vi "etlUSBClose.vi"(1 "lens":enum16{"0", "1"}(ring)) -> ()   [LabVIEW 2017]
uses:
  globalDevices.vi
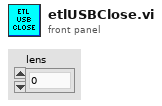
[diagram p1: front panel]
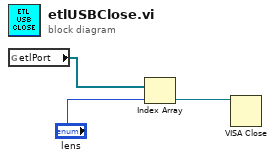
[diagram p0: block diagram]
diagram:
  n1 = global read "globalDevices.vi" "etlPort"() -> (w3:refnum<visa-resource-name>[])
  n2 = Index Array(array=w3, index="lens") -> (element=w1:refnum<visa-resource-name>)
  n3 = VISA Close(VISA resource name=w1) -> ()  [unwired: 1 in, 1 out]
